vi "exampleClient.vi"() -> ()   [LabVIEW 2017]
uses:
  <vilib>/httpClient/POSTBuffer.vi
  <vilib>/httpClient/LabVIEWHTTPClient.lvlib
panel:
  out "version":string
  in  "GetVersion":bool
  out "url":string
  in  "port":i32
  in  "ip":string
  out "response":string
  in  "Send":bool
  in  "Stop Button":bool
  in  "cmd":string
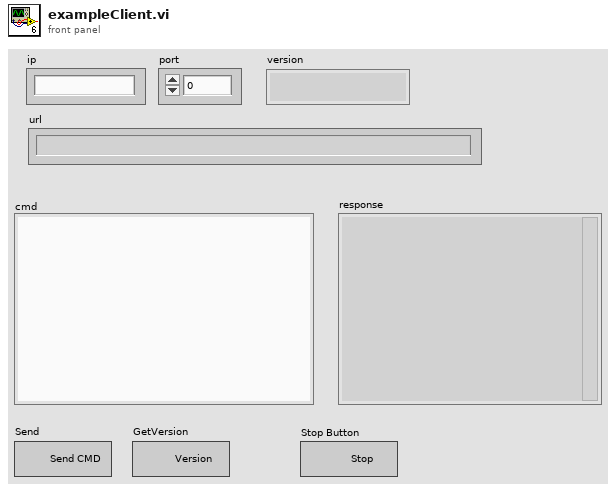
[diagram p1: front panel]
types:
  T1 = typedef "LabVIEWHTTPClient.lvlib/ClientHandle.ctl" = refnum<k1>
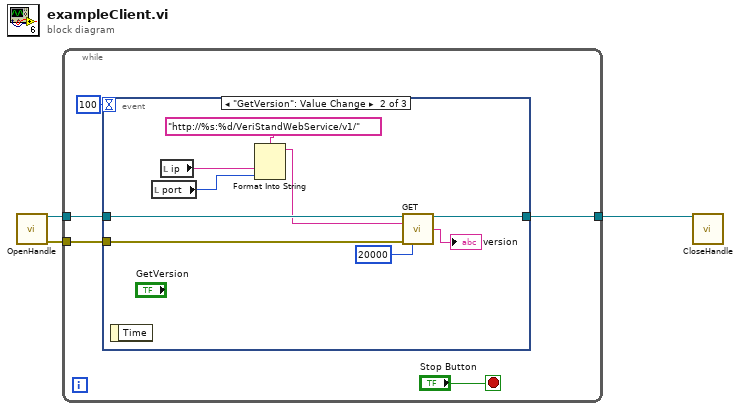
[diagram p0: block diagram]
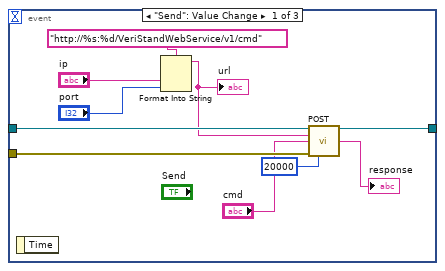
[diagram p2: hidden frame]
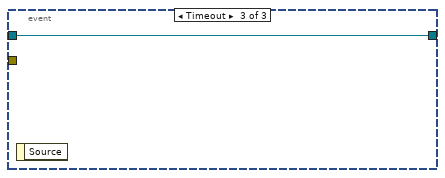
[diagram p3: hidden frame]
diagram:
  n1 = call <vilib>:"OpenHandle.vi"() -> ("client handle out"=w3:T1, "error out"=w2:errorcluster)  [unwired: 14 in]
  n2 = while {
    tunnel: w3 -> [w8]
    tunnel: w2 -> [w7]
    tunnel: [w6] -> w1
    stop <- "Stop Button" stop-if-true
    n3 = event shown="[1] \"GetVersion\": Value Change" {
      selector: _ -> [_ _ _]
      dyn-events: _ -> [_ _ _]
      timeout: 100 -> [_ _ _]
      tunnel: w8 -> [w18 w27 w28]
      tunnel: w7 -> [w17 w26 _]
      tunnel: [w15 w25 w28] -> w6
      event "Send": Value Change {
        n4 = event-data() -> ()  [unwired: 1 in, 1 out]
        n5 = Format Into String(format string="http://%s:%d/VeriStandWebService/v1/cmd" ("url"), "ip", "port") -> (resulting string=w9:string)  [unwired: 2 in, 1 out]
        "url" <- w9
        n6 = call-poly <vilib>:"POST.vi"("client handle"=w18, "url"=w9, "buffer"="cmd", "error in (no error)"=w17, "timeout (10000)"=20000) -> ("client handle out"=w15:T1, "body"=→"response":string)  [unwired: 7 in, 2 out]
      }
      event "GetVersion": Value Change {
        n7 = event-data() -> ()  [unwired: 1 in, 1 out]
        n8 = local read "port"() -> (w20:i32)
        n9 = local read "ip"() -> (w21:string)
        n10 = Format Into String(format string="http://%s:%d/VeriStandWebService/v1/" ("url"), w21, w20) -> (resulting string=w22:string)  [unwired: 2 in, 1 out]
        n11 = call <vilib>:"GET.vi"("client handle"=w27, "url"=w22, "error in (no error)"=w26, "timeout (10000)"=20000) -> ("client handle out"=w25:T1, "body"=→"version":string)  [unwired: 8 in, 2 out]
      }
      event Timeout {
        n12 = event-data() -> ()  [unwired: 1 in, 1 out]
      }
    }
  }
  n13 = call <vilib>:"CloseHandle.vi"("client handle"=w1) -> ()  [unwired: 14 in, 1 out]
